vi "Index Arrays - sv refnum.vi"(9 "Index array":u32[](array[numeric]), 11 "Array in":refnum<k21>[](array[refnum])) -> (3 "Array out":refnum<k21>[](array[refnum]))   [LabVIEW 2014]
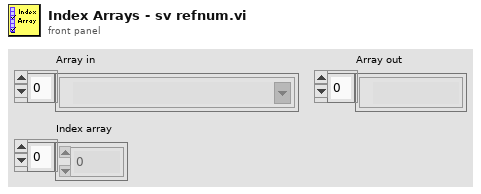
[diagram p1: front panel]
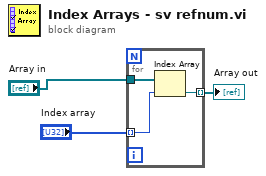
[diagram p0: block diagram]
diagram:
  n1 = for {
    tunnel: "Array in" -> [w6]
    tunnel: "Index array" -> [w5] mode=indexing
    tunnel: [w4] -> w1 mode=indexing
    n2 = Index Array(array=w6, index=w5) -> (element=w4:refnum<k21>)
  }
  "Array out" <- w1
